vi "sub_save-log.vi"(8 "error in":errorcluster, 10 "data":string, 11 "title":string) -> (0 "error out":errorcluster caption="erro out")   [LabVIEW 2016]
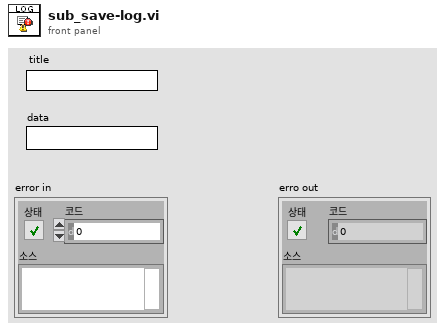
[diagram p1: front panel]
types:
  T1 = enum16{"open", "replace", "create", "open or create", "replace or create", "replace or create with confirmation"}
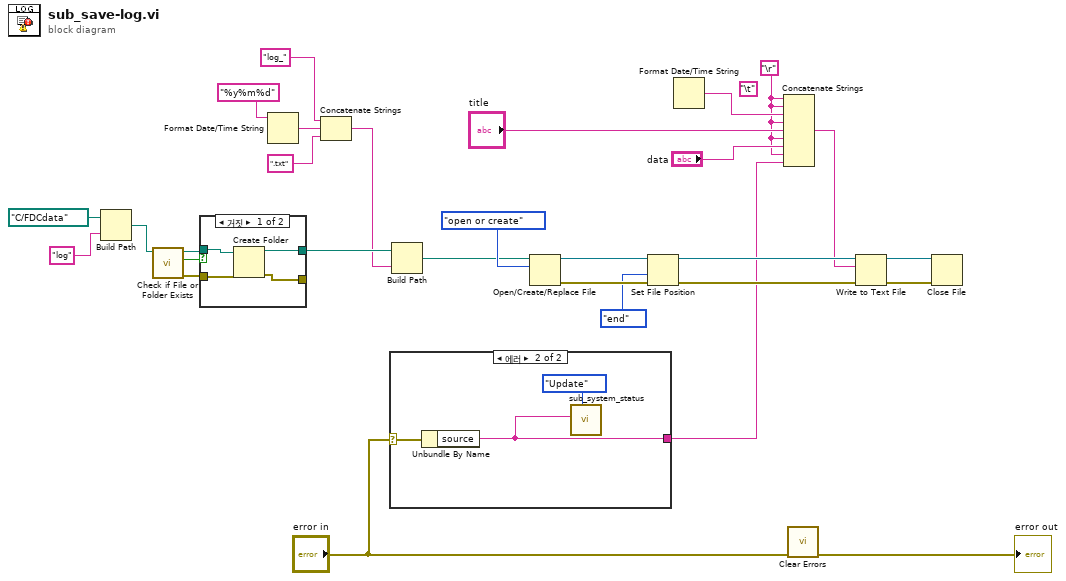
[diagram p0: block diagram]
diagram:
  (unwired) "\t"
  w3 = "\r"
  n1 = Build Path(base path=path "C:/FDCdata" ("베이스 경로"), name or relative path="log" ("이름 또는 상대 경로")) -> (appended path=w15:path)
  n2 = call <vilib>:"Check if File or Folder Exists.vi"("path"=w15) -> ("error out"=w19:errorcluster, "file or folder exists?"=w18:bool, "dup path"=w17:path)  [unwired: 8 in]
  n3 = case shown="거짓" w18 {
    tunnel: w17 -> [w33 w35]
    tunnel: w19 -> [w32 w34]
    tunnel: [w31 w35] -> w14
    tunnel: [w30 w34] -> _
    frame False {
      n4 = Create Folder(path (use dialog)=w33, error in=w32) -> (created path=w31:path, error out=w30:errorcluster)  [unwired: 1 in, 1 out]
    }
    frame True {
    }
  }
  n5 = Format Date/Time String(time format string (%c)="%y%m%d" ("시간 포맷 문자열 (%c)")) -> (date/time string=w9:string)  [unwired: 2 in]
  n6 = Concatenate Strings("log_" ("이름 또는 상대 경로"), w9, ".txt" ("문자열")) -> (w11:string)
  n7 = case shown="에러" "error in" {
    selector: "error in" -> [_ w38]
    tunnel: [_ w36] -> w20
    frame No Error {
    }
    frame Error {
      n8 = Unbundle By Name(w38) -> ("source"=w36:string)
      n9 = call "sub_system_status.vi"("Mode"=enum16{"Initial", "Update", "Clear"}."Update", "String in"=w36) -> ()  [unwired: 9 in, 1 out]
    }
  }
  n10 = Build Path(base path=w14, name or relative path=w11) -> (appended path=w7:path)
  n11 = Open/Create/Replace File(file path (use dialog)=w7, operation (0:open)=T1."open or create" ("동작(0:open)")) -> (refnum out=w24:refnum<file>, error out=w26:errorcluster)  [unwired: 4 in, 1 out]
  n12 = Set File Position(refnum=w24, from (0:start)=enum16{"start", "end", "current"}."end" ("시작(0:시작)"), error in=w26) -> (refnum out=w23:refnum<file>, error out=w25:errorcluster)  [unwired: 1 in]
  n13 = Format Date/Time String() -> (date/time string=w5:string)  [unwired: 3 in]
  n14 = Concatenate Strings(w3, w3, w5, w3, "title", w3, "data", w3, w20) -> (w21:string)
  n15 = call <vilib>:"Clear Errors.vi"("error in (no error)"="error in") -> ("error out"=→"error out":errorcluster)  [unwired: 5 in, 1 out]
  n16 = Write to Text File(file (use dialog)=w23, text=w21, error in=w25) -> (refnum out=w28:refnum<file>, error out=w29:errorcluster)  [unwired: 1 in, 1 out]
  n17 = Close File(refnum=w28, error in=w29) -> ()  [unwired: 2 out]
